vi "DSF.Transceiver.UDP.Get Max Buffer Size.vi"(11 "UDP Transceiver in":refnum<class "DSF.Transceiver.UDP.lvclass">=refnum) -> (2 "max buffer size":u64 format="%d bytes", 3 "UDP Transceiver out":refnum<class "DSF.Transceiver.UDP.lvclass">)   [LabVIEW 2017, in "DSF.Transceiver.UDP.lvlib" / "DSF.Transceiver.UDP.lvclass"]
uses:
  DSF.Transceiver.UDP.lvclass
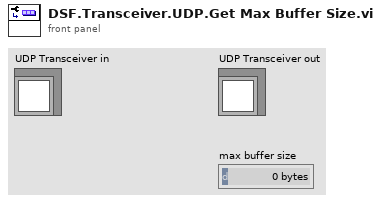
[diagram p1: front panel]
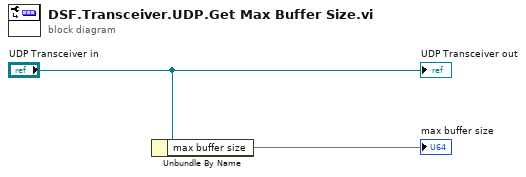
[diagram p0: block diagram]
diagram:
  n1 = Unbundle By Name("UDP Transceiver in") -> ("max buffer size"=→"max buffer size")
  "UDP Transceiver out" <- "UDP Transceiver in"
